vi "init.vi"(8 "error in (no error)":errorcluster, 11 "ComicVine_manager in":refnum<class "ComicVine_manager.lvclass">) -> (0 "error out":errorcluster, 3 "ComicVine_manager out":refnum<class "ComicVine_manager.lvclass">)   [LabVIEW 2024, in "ComicVine_manager.lvclass"]
uses:
  ComicVine_manager.lvclass
  states--enum.ctl
  ComicVine_manager.lvclass/ComicVine_manager.ctl
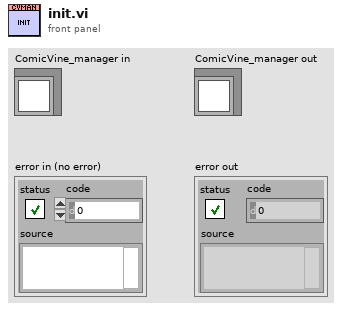
[diagram p1: front panel]
types:
  T1 = typedef "ComicVine_manager.lvclass/states--enum.ctl" = enum16{"start", "running", "start timer", "update file", "set directories", "wait", "shutdown"}
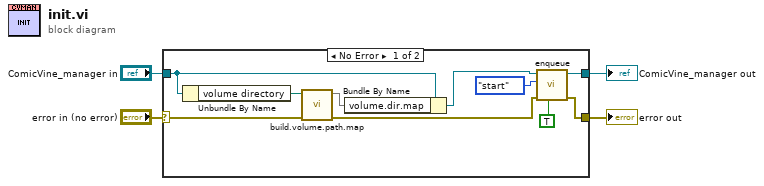
[diagram p0: block diagram]
diagram:
  n1 = case shown="No Error" "error in (no error)" {
    selector: "error in (no error)" -> [w12 w16]
    tunnel: [w8 w16] -> w3
    tunnel: [w11 w15] -> w1
    tunnel: "ComicVine_manager in" -> [w10 w15]
    frame No Error {
      n2 = Unbundle By Name(w10) -> ("volume directory"=w14:path)
      n3 = call "build.volume.path.map"("error in (no error)"=w12, "Folder Path"=w14) -> ("error out"=w9:errorcluster, "map"=w13:map{i32, path})  [unwired: 8 in]
      n4 = Bundle By Name(cluster=w10, "volume.dir.map"=w13) -> (w5:refnum<class "ComicVine_manager.lvclass">)
      n5 = call "enqueue.vi"("priority (f)"=TRUE, "error in (no error)"=w9, "cmd"=states--enum."start", "ComicVine_manager in"=w5) -> ("error out"=w8:errorcluster, "ComicVine_manager out"=w11:refnum<class "ComicVine_manager.lvclass">)  [unwired: 6 in]
    }
    frame Error {
    }
  }
  "error out" <- w3
  "ComicVine_manager out" <- w1
